vi "Sum of N Gaussians with offseat fit_MODCA.vi"(7 "Data X":dbl[](array[numeric]), 8 "number of peaks":i32=3, 9 "Intensities":dbl[](array[numeric]), 10 "Energies":dbl[](array[numeric]), 11 "Data Y":dbl[](array[numeric])) -> (1 "Sum of N Gaussians":cluster{cdb[]}[](graph), 3 "Parameters Fitted":dbl[][](array[numeric]))   [LabVIEW 2020]
doc: "Demonstrates fitting data to a model that is the sum of three Gaussian curves and an offset."
uses:
  0ea831b5-f57b-8c4c-a27d-8b741b9c5071.vi
  da65fc18-1473-244d-89c7-39926d06bfb6.vi
  <vilib>/Utility/Data Type/Get Array Information.vi
  <vilib>/Utility/Data Type/Get Type Information.vi
  <vilib>/gmath/NumericalOptimization/Nonlinear Curve Fit LM.vi
  <vilib>/gmath/NI_Gmath.lvlib
panel:
  out "appended array":dbl[][](array[numeric])
  out "Data Out":dbl[][](array[numeric])
  out "Intensity Centroids":dbl[](array[numeric])
  out "Fitted Peaks - Centroids":dbl[](array[numeric])
  out "Auto Guess":dbl[](array[numeric])
  out "Fit A - mu - Sigma":dbl[][](array[numeric])
  out "Number of function calls":i32
  out "Residue":dbl
  out "DC offset fit":dbl
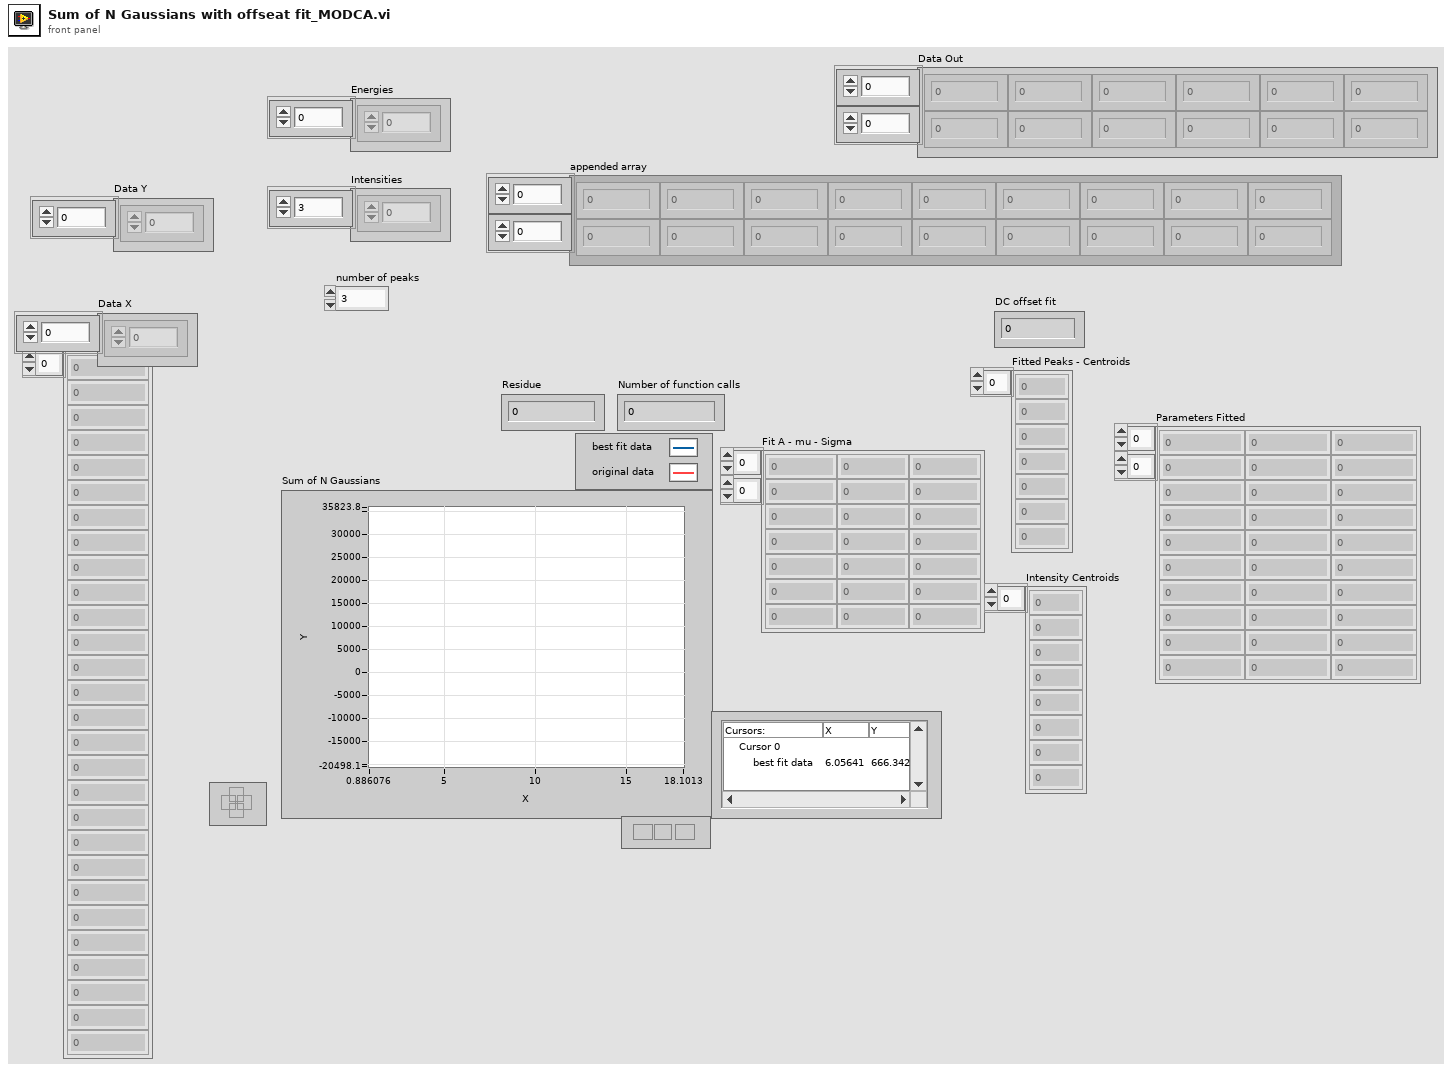
[diagram p1: front panel]
types:
  T1 = cluster{"Numeric Control":dbl, "Numeric Control":dbl}
  T2 = cluster{"Numeric Control":dbl, "Numeric Control":dbl}[]
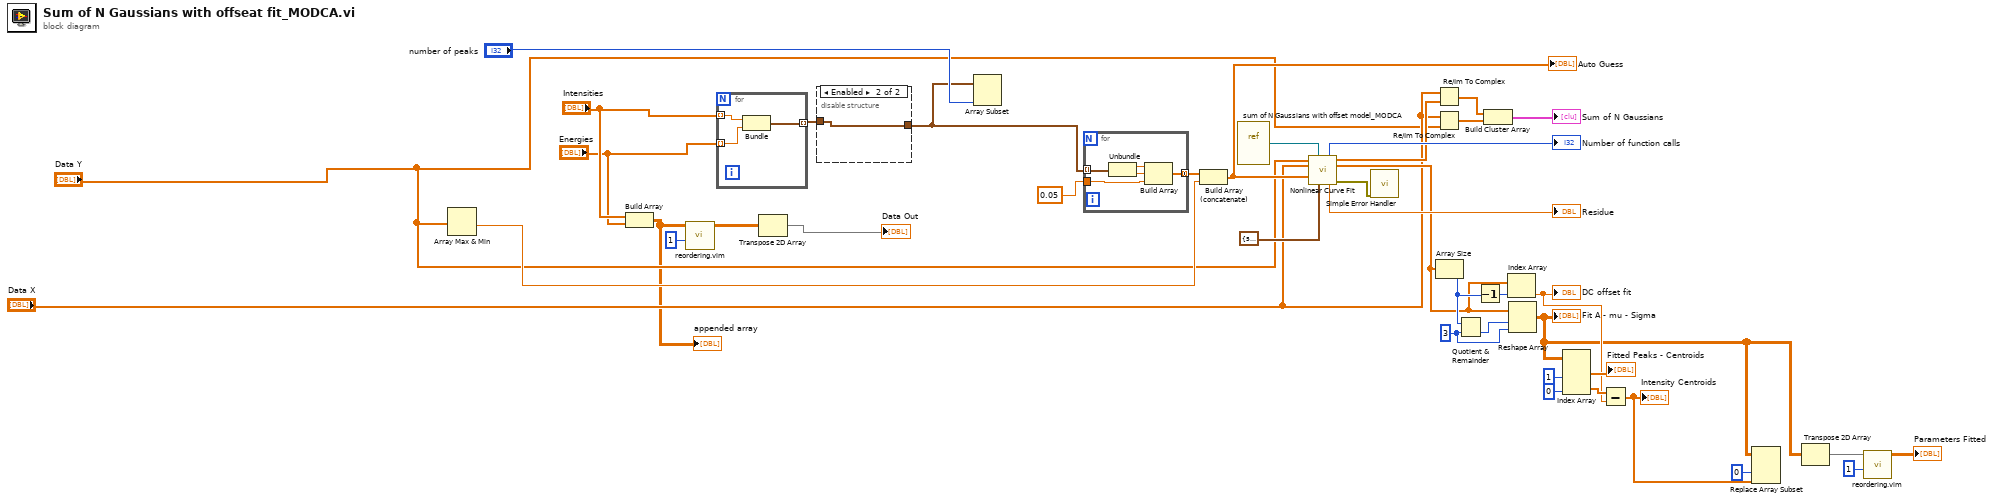
[diagram p0: block diagram]
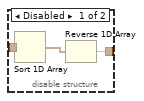
[diagram p2: hidden frame]
diagram:
  w26 = 3 ("y")
  n1 = Array Max & Min(array="Data Y") -> (min value=w15:dbl)  [unwired: 3 out]
  n2 = Build Array("Intensities", "Energies") -> (w3:dbl[][])
  "appended array" <- w3
  n3 = call "reordering.vim"("Row to Reorder"=1, "Data In"=w3) -> ("Data Out"=w2:dbl[][])  [unwired: 8 in, 1 out]
  n4 = for {
    tunnel: "Intensities" -> [w43] mode=indexing
    tunnel: "Energies" -> [w42] mode=indexing
    tunnel: [w41] -> w18 mode=indexing
    n5 = Bundle("Numeric Control"=w43, "Numeric Control"=w42) -> (w41:T1)  [unwired: 1 in]
  }
  n6 = Transpose 2D Array(2D array=w2) -> (transposed array=→"Data Out":dbl[][])
  n7 = disable-structure shown="Enabled" {
    disable-tunnel: w18 -> [w46 w47]
    disable-tunnel: [w44 w47] -> w16
    frame Disabled {
      n8 = Sort 1D Array(array=w46) -> (sorted array=w45:T2)
      n9 = Reverse 1D Array(array=w45) -> (reversed array=w44:T2)
    }
    frame Enabled {
    }
  }
  n10 = Array Subset(array=w16, length="number of peaks") -> ()  [unwired: 1 in, 1 out]
  n11 = for {
    tunnel: w16 -> [w52] mode=indexing
    tunnel: [w49] -> w31 mode=concatenating
    tunnel: 0.05 -> [w48]
    n12 = Unbundle(w52) -> ("Numeric Control"=w51:dbl, "Numeric Control"=w50:dbl)
    n13 = Build Array(w51, w50, w48) -> (w49:dbl[])
  }
  n14 = Build Array (concatenate)(w31, w15) -> (w34:dbl[])
  "Auto Guess" <- w34
  n15 = vi-ref "sum of N Gaussians with offset model_MODCA.vi"() -> (w32:refnum<vi>)
  n16 = call-poly <vilib>:"Nonlinear Curve Fit.vi"("Y"="Data Y", "f(x,a)"=w32, "X"="Data X", "initial parameters"=w34, "termination"=cluster{"max iteration":i32, "tolerance":dbl} {"max iteration"=500, "tolerance"=1e-07}) -> ("number of function calls"=→"Number of function calls":i32, "best nonlinear fit"=w39:dbl[], "best fit parameters"=w29:dbl[], "residue"=→"Residue":dbl, "error out"=w33:errorcluster)  [unwired: 5 in, 1 out]
  n17 = call <vilib>:"Simple Error Handler.vi"("error in (no error)"=w33) -> ()  [unwired: 4 in, 5 out]
  n18 = Re/Im To Complex(1:w39, 2:"Data X") -> (0:w35:cdb[])
  n19 = Re/Im To Complex(1:"Data Y", 2:"Data X") -> (0:w36:cdb[])
  n20 = Array Size(array=w29) -> (size(s)=w30:i32)
  n21 = Quotient & Remainder(x=w30, y=w26) -> (floor(x/y)=w27:i32)  [unwired: 1 out]
  n22 = Decrement(x=w30) -> (x-1=w28:i32)
  n23 = Build Cluster Array(w35, w36) -> (→"Sum of N Gaussians":cluster{cdb[]}[])
  n24 = Index Array(array=w29, index=w28) -> (element=w19:dbl)
  "DC offset fit" <- w19
  n25 = Reshape Array(w29, w27, w26) -> (w7:dbl[][])
  "Fit A - mu - Sigma" <- w7
  n26 = Index Array(array=w7, index (col) #1=1 ("disabled index (col)"), index (col) #2=0 ("index (col)")) -> (element #1=→"Fitted Peaks - Centroids":dbl[], element #2=w20:dbl[])  [unwired: 2 in]
  n27 = Subtract(x=w20, y=w19) -> (x-y=w12:dbl[])
  "Intensity Centroids" <- w12
  n28 = Replace Array Subset(array=w7, new element=w12, index (col)=0 ("disabled index (col)")) -> ()  [unwired: 1 in, 1 out]
  n29 = Transpose 2D Array(2D array=w7) -> (transposed array=w8:dbl[][])
  n30 = call "reordering.vim"("Row to Reorder"=1, "Data In"=w8) -> ("Data Out"=→"Parameters Fitted":dbl[][])  [unwired: 8 in, 1 out]
